vi "Demo_comm_setting.vi"(8 "error in":errorcluster) -> (0 "error out":errorcluster, 1 "Ignore IsActive":cluster{"Count on Breakdown?":bool}, 2 "Card Numbers":cluster{"CID":string[]}, 3 "Comm Setting":T1)   [LabVIEW 2017]
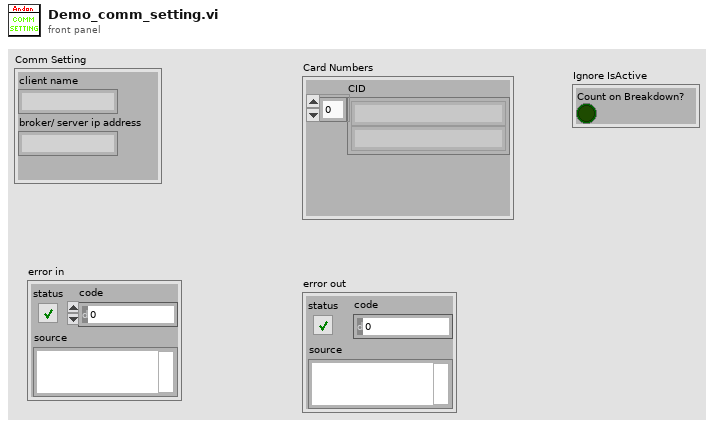
[diagram p1: front panel]
types:
  T1 = cluster{"client name":string, "broker/ server ip address":string}
  T2 = enum32{"invalid app kind", "Development System", "Run Time System", "Student Edition", "Embedded LabVIEW", "Evaluation", "Custom"}
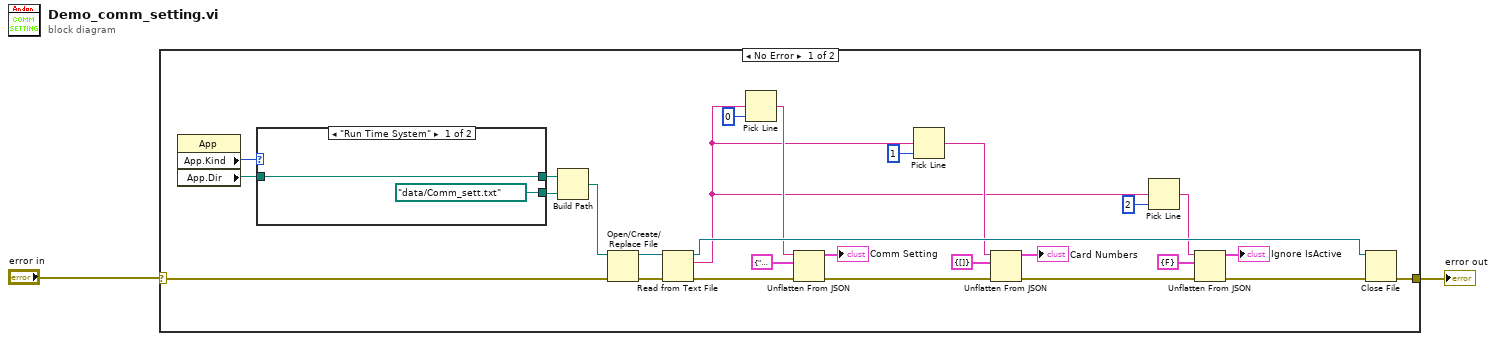
[diagram p0: block diagram]
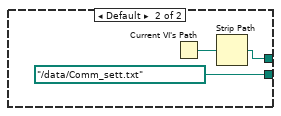
[diagram p2: hidden frame]
diagram:
  n1 = case shown="No Error" "error in" {
    selector: "error in" -> [w22 w35]
    tunnel: [w18 w35] -> w1
    frame No Error {
      n2 = property class="App"() -> ("App.Kind"=w29:T2, "App.Dir"=w28:path)  [unwired: 2 in, 2 out]
      n3 = case shown="\"Run Time System\"" w29 {
        tunnel: w28 -> [w31 _]
        tunnel: [path "data/Comm_sett.txt" ("path") path "../data/Comm_sett.txt" ("path")] -> w26
        tunnel: [w31 w32] -> w25
        frame "Run Time System" {
        }
        frame Default {
          n4 = Current VI's Path() -> (path=w33:path)
          n5 = Strip Path(path=w33) -> (stripped path=w32:path)  [unwired: 1 out]
        }
      }
      n6 = Build Path(base path=w25, name or relative path=w26) -> (appended path=w27:path)
      n7 = Open/Create/Replace File(file path (use dialog)=w27, error in=w22) -> (refnum out=w24:refnum<file>, error out=w23:errorcluster)  [unwired: 4 in, 1 out]
      n8 = Read from Text File(file (use dialog)=w24, error in=w23) -> (refnum out=w19:refnum<file>, text=w3:string, error out=w20:errorcluster)  [unwired: 2 in, 1 out]
      n9 = Pick Line(multi-line string=w3, line index=0) -> (output string=w16:string)  [unwired: 1 in]
      n10 = Unflatten From JSON(JSON string=w16, type and defaults=T1 {"client name"="", "broker/ server ip address"=""}, error in (no error)=w20) -> (value=→"Comm Setting":T1, error out=w13:errorcluster)  [unwired: 4 in]
      n11 = Pick Line(multi-line string=w3, line index=1) -> (output string=w12:string)  [unwired: 1 in]
      n12 = Unflatten From JSON(JSON string=w12, type and defaults=cluster{"CID":string[]} {"CID"=[]}, error in (no error)=w13) -> (value=→"Card Numbers":cluster{"CID":string[]}, error out=w7:errorcluster)  [unwired: 4 in]
      n13 = Pick Line(multi-line string=w3, line index=2) -> (output string=w9:string)  [unwired: 1 in]
      n14 = Unflatten From JSON(JSON string=w9, type and defaults=cluster{"Count on Breakdown?":bool} {"Count on Breakdown?"=FALSE} ("Cluster 2"), error in (no error)=w7) -> (value=→"Ignore IsActive":cluster{"Count on Breakdown?":bool}, error out=w6:errorcluster)  [unwired: 4 in]
      n15 = Close File(refnum=w19, error in=w6) -> (error out=w18:errorcluster)  [unwired: 1 out]
    }
    frame Error {
    }
  }
  "error out" <- w1
